vi "Sequence RPM in Range.vi"(1 "Actual RPM":i16, 2 "Target RPM":i16) -> (0 "In Range?":bool)   [LabVIEW 2024, in "Auto Modo.lvlib"]
uses:
  Auto Modo.lvlib
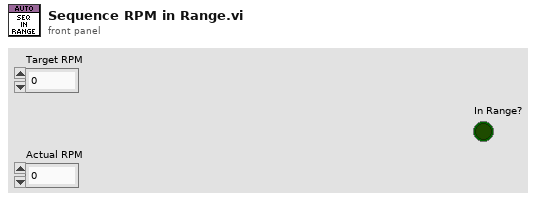
[diagram p1: front panel]
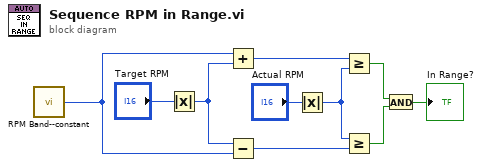
[diagram p0: block diagram]
diagram:
  n1 = call "RPM Band--constant.vi"() -> ("RPM Band"=w9:i16)  [unwired: 1 in]
  n2 = Absolute Value(x="Target RPM") -> (abs(x)=w8:i16)
  n3 = Add(x=w9, y=w8) -> (x+y=w6:i16)
  n4 = Subtract(x=w8, y=w9) -> (x-y=w4:i16)
  n5 = Absolute Value(x="Actual RPM") -> (abs(x)=w5:i16)
  n6 = Greater Or Equal?(x=w6, y=w5) -> (x >= y?=w3:bool)
  n7 = Greater Or Equal?(x=w5, y=w4) -> (x >= y?=w2:bool)
  n8 = And(x=w3, y=w2) -> (x .and. y?=→"In Range?":bool)
